vi "Scale.vi"(9 "Waveform Data":dbl[](array[numeric])) -> (1 "Scaled Waveform Data":u16[](array[numeric]))   [LabVIEW 2013, in "Tektronix AFG 3000 Series.lvlib"]
doc: "This VI scales a data array so that the maximum (positive or negative) value in the array corresponds to the maximum allowed value (positive or negative) for the instrument."
uses:
  Tektronix AFG 3000 Series.lvlib
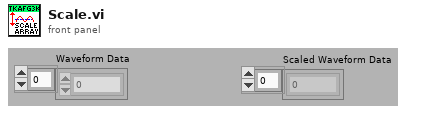
[diagram p1: front panel]
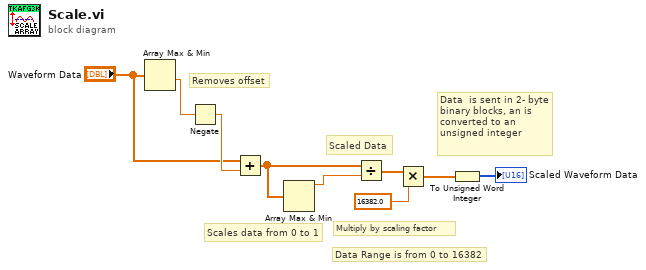
[diagram p0: block diagram]
diagram:
  # "Data  is sent in 2- byte binary blocks, an is converted to an unsigned integer"
  # "Multiply by scaling factor"
  # "Scaled Data"
  # "Scales data from 0 to 1"
  # "Removes offset"
  # "Data Range is from 0 to 16382"
  n1 = Array Max & Min(array="Waveform Data") -> (min value=w8:dbl)  [unwired: 3 out]
  n2 = Negate(x=w8) -> (-x=w9:dbl)
  n3 = Add(x="Waveform Data", y=w9) -> (x+y=w5:dbl[])
  n4 = Array Max & Min(array=w5) -> (max value=w6:dbl)  [unwired: 3 out]
  n5 = Divide(x=w5, y=w6) -> (x/y=w4:dbl[])
  n6 = Multiply(x=w4, y=16382.0) -> (x*y=w2:dbl[])
  n7 = To Unsigned Word Integer(number=w2) -> (unsigned 16bit integer=→"Scaled Waveform Data":u16[])
